vi "Load program.vi"(8 "error in":errorcluster) -> (0 "error out":errorcluster, 2 "Zone Setup Array Data":T1)   [LabVIEW 2019]
uses:
  Controls/Zone Setup Array.ctl
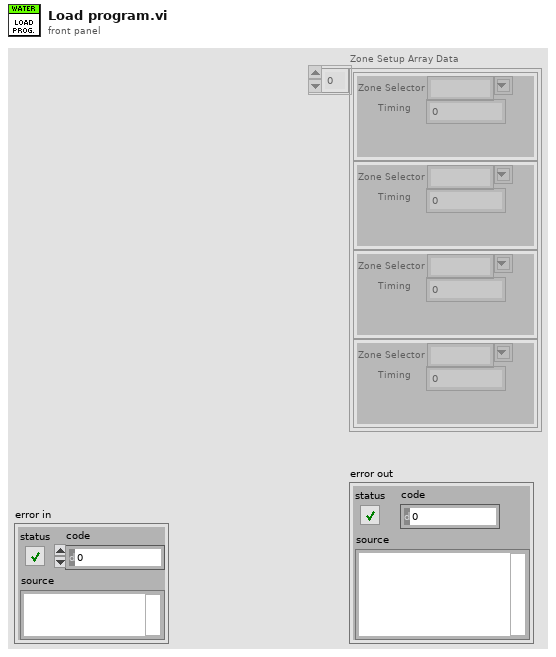
[diagram p1: front panel]
types:
  T1 = typedef "Zone Setup Array.ctl" = cluster{"Zone Selector":string, "Timing":dbl}[]
  T2 = enum16{"open", "replace", "create", "open or create", "replace or create", "replace or create with confirmation"}
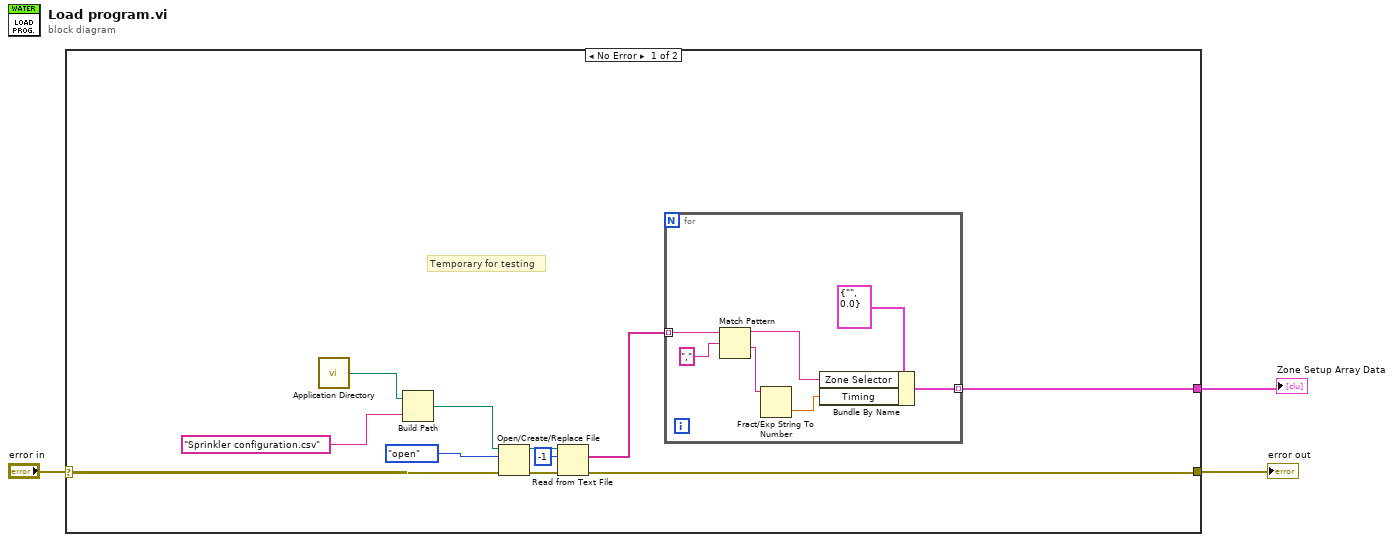
[diagram p0: block diagram]
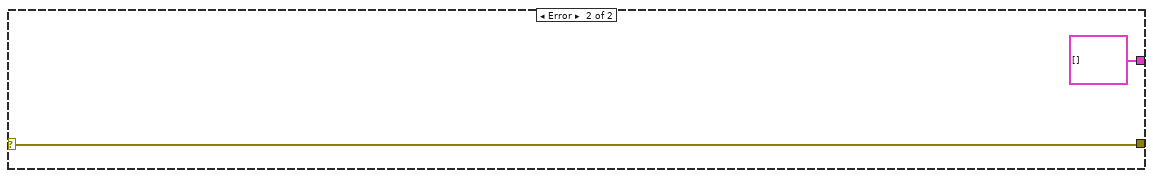
[diagram p2: hidden frame]
diagram:
  n1 = case shown="No Error" "error in" {
    selector: "error in" -> [w10 w23]
    tunnel: [w8 w23] -> w2
    tunnel: [w5 cluster{"Zone Selector":string, "Timing":dbl}[] []] -> w1
    frame No Error {
      # "Temporary for testing"
      n2 = call <vilib>:"Application Directory.vi"() -> ("Application Directory"=w9:path)
      n3 = Build Path(base path=w9, name or relative path="Sprinkler configuration.csv") -> (appended path=w4:path)
      n4 = Open/Create/Replace File(file path (use dialog)=w4, error in=w10, operation (0:open)=T2."open") -> (refnum out=w12:refnum<file>, error out=w11:errorcluster)  [unwired: 3 in, 1 out]
      n5 = Read from Text File(file (use dialog)=w12, count=-1, error in=w11) -> (text=w7:string[], error out=w8:errorcluster)  [unwired: 1 in, 2 out]
      n6 = for {
        tunnel: w7 -> [w21] mode=indexing
        tunnel: [w15] -> w5 mode=indexing
        n7 = Match Pattern(string=w21, regular expression=",") -> (before substring=w18:string, after substring=w17:string)  [unwired: 1 in, 2 out]
        n8 = Fract/Exp String To Number(string=w17) -> (number=w16:dbl)  [unwired: 3 in, 1 out]
        n9 = Bundle By Name(cluster=cluster{"Zone Selector":string, "Timing":dbl} {"Zone Selector"="", "Timing"=0.0} ("Zone Selector"), "Zone Selector"=w18, "Timing"=w16) -> (w15:cluster{"Zone Selector":string, "Timing":dbl})
      }
    }
    frame Error {
    }
  }
  "error out" <- w2
  "Zone Setup Array Data" <- w1
